vi "SP Append Filter Skirt Limit Waveform.vi"(4 "Limit Format":T2, 5 "Number of Points":i32, 6 "Measured Parameter":T3={"Stimulus Port"=1, "Response Port"=1} {"Stimulus Port" min=1 step=1; "Response Port" min=1 step=1}, 7 "Attribute Name (NI_ChannelName)":string="NI_ChannelName", 8 "error in (no error)":errorcluster, 9 "Limits Pass/Fail":cluster{"Upper Pass?":bool, "Lower Pass?":bool}, 10 "Upper and Lower Limits":T1={"Upper Limit"={"F0"=500.0, "dF"=1.0, "Formatted Values"=[-6.0, -6.0, -6.0, -6.0, -6.0, -6.0, -5.0, -4.0, -3.0, -2.0, -1.0017226002993769, -0.8636286738753696, -1.012432061728755, -0.8135188671805874, -1.084383696215112, -1.192695586219516, -0.8228939725524264, -1.1588169801015764, -1.0069715761898415, -0.8118111488159718, -0.9516999033989667, -1.0842662636672022, -1.0261931083967077, -0.816874162233468, -0.8335770068326294, -1.1794529347576463, -1.1032959879886735, -1.197742447623333, -0.9631229100196212, -0.9908453124177325, -0.9835470980893588, -1.10217991844936, -0.8956607286257672, -0.8794782872077156, -0.9013683651609963, -1.0772188731817596, -0.992723355191172, -0.9536275499498994, -0.9874327685983141, -0.921963653527827, -0.8848787728556787, -1.1874980208218, -0.996957511881206, -0.9972503730309241, -0.8866139538542095, -1.07344181331393, -0.881559772443858, -1.0112449407130875, -0.9865384477979471, -0.9901446738263366, -1.1718630063784758, -0.9951725256878827, -0.931778781153855, -0.9846289731021831, -0.851763264124267, -0.9086965469391421, -0.8349429101974368, -0.8383742350256687, -1.106571816484691, -0.9554005266395742, -0.9376822403043366, -1.131287512516927, -1.0382288806403288, -0.917054052988136, -0.9489467877812984, -0.9264227759143271, -1.0918690925892351, -1.1668737446636852, -1.0021735712381068, -1.1541225361979714, -1.1931131329605709, -0.8730502330378824, -0.850411285659811, -1.137775166801135, -1.1870586525662095, -1.0926571181161528, -1.118993526927924, -1.1211410787283602, -0.8920697041785735, -0.888430731015914, -1.0656600076605476, -1.1666787859795846, -1.0713340188424678, -0.8625910088884297, -1.1434360227216422, -0.9217710376784376, -1.1218396445954617, -0.9558195687190933, -1.1773692443654946, -1.0827782751424972, -1.1567791336122029, -0.8684407402614696, -0.8177845157195978, -0.9040657051180614, -0.9313557288389804, -1.0236831450620423, -1.050426714979035, -0.8344777069605718, -0.8274082929927138, -1.1990080831766776, -1.0947798998491134, -1.1963114865246718, -1.0016247375583676, -1.0877110100652403, -1.1556028882288836, -1.1918380581525247, -0.9751292214691399, -0.8884133044813358, -1.0347444321214612, -0.9445125246491541, -2.0, -3.0, -4.0, -5.0, -6.0, -6.0, -6.0, -6.0, -6.0, -6.0]}, "Lower Limit"={"F0"=500.0, "dF"=1.0, "Formatted Values"=[-6.0, -6.0, -6.0, -6.0, -6.0, -6.0, -5.0, -4.0, -3.0, -2.0, -1.0017226002993769, -0.8636286738753696, -1.012432061728755, -0.8135188671805874, -1.084383696215112, -1.192695586219516, -0.8228939725524264, -1.1588169801015764, -1.0069715761898415, -0.8118111488159718, -0.9516999033989667, -1.0842662636672022, -1.0261931083967077, -0.816874162233468, -0.8335770068326294, -1.1794529347576463, -1.1032959879886735, -1.197742447623333, -0.9631229100196212, -0.9908453124177325, -0.9835470980893588, -1.10217991844936, -0.8956607286257672, -0.8794782872077156, -0.9013683651609963, -1.0772188731817596, -0.992723355191172, -0.9536275499498994, -0.9874327685983141, -0.921963653527827, -0.8848787728556787, -1.1874980208218, -0.996957511881206, -0.9972503730309241, -0.8866139538542095, -1.07344181331393, -0.881559772443858, -1.0112449407130875, -0.9865384477979471, -0.9901446738263366, -1.1718630063784758, -0.9951725256878827, -0.931778781153855, -0.9846289731021831, -0.851763264124267, -0.9086965469391421, -0.8349429101974368, -0.8383742350256687, -1.106571816484691, -0.9554005266395742, -0.9376822403043366, -1.131287512516927, -1.0382288806403288, -0.917054052988136, -0.9489467877812984, -0.9264227759143271, -1.0918690925892351, -1.1668737446636852, -1.0021735712381068, -1.1541225361979714, -1.1931131329605709, -0.8730502330378824, -0.850411285659811, -1.137775166801135, -1.1870586525662095, -1.0926571181161528, -1.118993526927924, -1.1211410787283602, -0.8920697041785735, -0.888430731015914, -1.0656600076605476, -1.1666787859795846, -1.0713340188424678, -0.8625910088884297, -1.1434360227216422, -0.9217710376784376, -1.1218396445954617, -0.9558195687190933, -1.1773692443654946, -1.0827782751424972, -1.1567791336122029, -0.8684407402614696, -0.8177845157195978, -0.9040657051180614, -0.9313557288389804, -1.0236831450620423, -1.050426714979035, -0.8344777069605718, -0.8274082929927138, -1.1990080831766776, -1.0947798998491134, -1.1963114865246718, -1.0016247375583676, -1.0877110100652403, -1.1556028882288836, -1.1918380581525247, -0.9751292214691399, -0.8884133044813358, -1.0347444321214612, -0.9445125246491541, -2.0, -3.0, -4.0, -5.0, -6.0, -6.0, -6.0, -6.0, -6.0, -6.0]}}, 11 "Waveforms in":waveform(dbl)[](array[waveform])) -> (0 "error out":errorcluster, 3 "Waveforms out":waveform(dbl)[](array[waveform]))   [LabVIEW 2011]
uses:
  TypeDefs/SP Parameter.ctl
  TypeDefs/SP Format.ctl
  TypeDefs/SP Channel Type.ctl
  Channel Test Status Enumeration.ctl
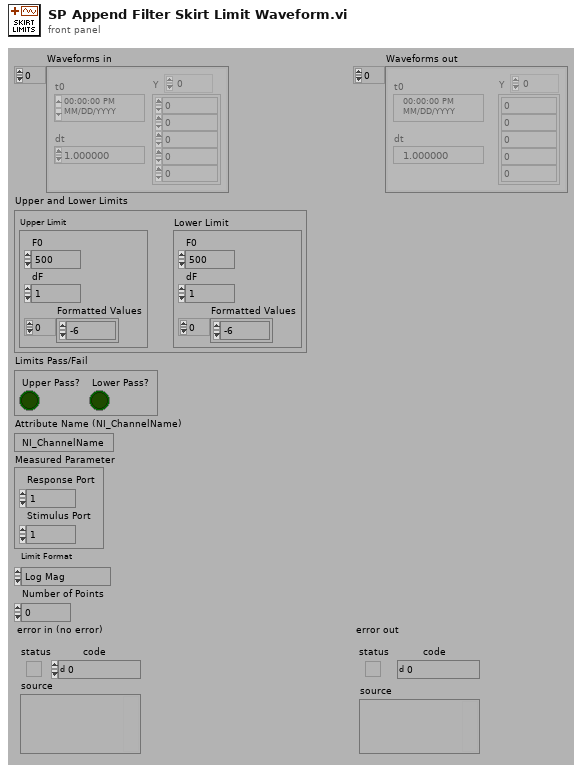
[diagram p1: front panel]
types:
  T1 = cluster{"Upper Limit":cluster{"F0":dbl, "dF":dbl, "Formatted Values":dbl[]}, "Lower Limit":cluster{"F0":dbl, "dF":dbl, "Formatted Values":dbl[]}}
  T2 = typedef "SP Format.ctl" = enum16{"Log Mag", "Lin Mag", "SWR", "Phase", "Expanded Phase", "Delay", "Insertion Loss", "Isolation", "Return Loss"}
  T3 = typedef "SP Parameter.ctl" = cluster{"Stimulus Port":i8, "Response Port":i8}
  T4 = typedef "SP Channel Type.ctl" = enum16{"Frequency", "Data", "Limit", "Adapter", "Memory", "Value", "Value Limit"}
  T5 = typedef "Channel Test Status Enumeration.ctl" = enum16{"Fail", "Pass", "Abort", "Error", "Done", "Pass by Sample", "Fail by Sample", "Pass Override", "Fail Override", "Not Tested"}
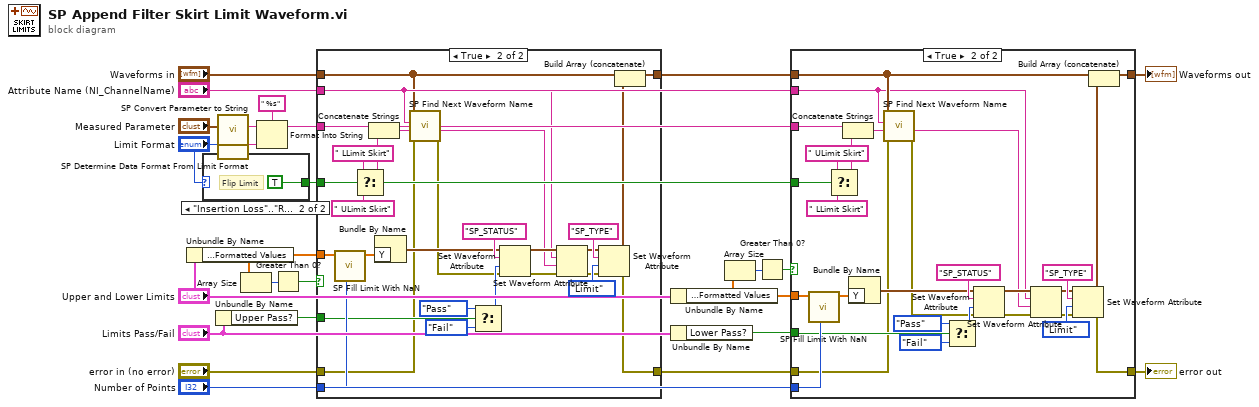
[diagram p0: block diagram]
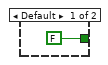
[diagram p3: hidden frame]
diagram:
  n1 = Unbundle By Name("Upper and Lower Limits") -> ("Upper Limit.Formatted Values"=w12:dbl[])
  n2 = case shown="\"Insertion Loss\"..\"Return Loss\"" "Limit Format" {
    tunnel: [FALSE TRUE] -> w9
    frame Default {
    }
    frame "Insertion Loss".."Return Loss" {
      # "Flip Limit"
    }
  }
  n3 = Unbundle By Name("Limits Pass/Fail") -> ("Upper Pass?"=w18:bool)
  n4 = call "SP Convert Parameter to String.vi"("Parameter"="Measured Parameter") -> ("Parameter String"=w15:string)  [unwired: 10 out]
  n5 = call "SP Determine Data Format From Limit Format.vi"("Limit Format"="Limit Format") -> ("Format String"=w14:string)
  n6 = Array Size(array=w12) -> (size(s)=w23:i32)
  n7 = Format Into String(format string=" %s", initial string=w15, w14) -> (resulting string=w10:string)  [unwired: 1 in, 1 out]
  n8 = Greater Than 0?(x=w23) -> (x > 0?=w21:bool)
  n9 = case shown="True" w21 {
    tunnel: "Waveforms in" -> [w28 w35]
    tunnel: "error in (no error)" -> [w29 w31]
    tunnel: [w29 w38] -> w4
    tunnel: "Attribute Name (NI_ChannelName)" -> [_ w33]
    tunnel: w12 -> [_ w53]
    tunnel: w10 -> [_ w58]
    tunnel: [w28 w36] -> w3
    tunnel: w18 -> [_ w47]
    tunnel: w9 -> [_ w54]
    tunnel: "Number of Points" -> [_ w51]
    frame False {
    }
    frame True {
      n10 = call "SP Fill Limit With NaN.vi"("Number of Points"=w51, "Limit"=w53) -> ("Filled Limit"=w52:dbl[])  [unwired: 9 out]
      n11 = Select(t=" LLimit Skirt", s=w54, f=" ULimit Skirt") -> (s? t:f=w55:string)
      n12 = Concatenate Strings(w58, w55) -> (w34:string)
      n13 = Bundle By Name("Y"=w52) -> (w45:waveform(dbl))  [unwired: 1 out]
      n14 = call "SP Find Next Waveform Name.vi"("error in (no error)"=w31, "Prospective Base Name"=w34, "Attribute Name (NI_ChannelName)"=w33, "Waveforms in"=w35) -> ("error out"=w30:errorcluster, "Channel Name"=w32:string)  [unwired: 6 in]
      n15 = Select(t=Channel_Test_Status_Enumeration."Pass" ("Channel Status Enumeration"), s=w47, f=Channel_Test_Status_Enumeration."Fail" ("Channel Status Enumeration")) -> (s? t:f=w46:T5)
      n16 = Set Waveform Attribute(4:w30, 5:w46, 6:"SP_STATUS", 7:w45) -> (0:w39:errorcluster, 3:w42:waveform(dbl))  [unwired: 1 out]
      n17 = Set Waveform Attribute(4:w39, 5:w32, 6:w33, 7:w42) -> (0:w40:errorcluster, 3:w41:waveform(dbl))  [unwired: 1 out]
      n18 = Set Waveform Attribute(4:w40, 5:SP_Channel_Type."Limit" ("Channel Type"), 6:"SP_TYPE", 7:w41) -> (0:w38:errorcluster, 3:w37:waveform(dbl))  [unwired: 1 out]
      n19 = Build Array (concatenate)(w35, w37) -> (w36:waveform(dbl)[])
    }
  }
  n20 = Unbundle By Name("Upper and Lower Limits") -> ("Lower Limit.Formatted Values"=w6:dbl[])
  n21 = Unbundle By Name("Limits Pass/Fail") -> ("Lower Pass?"=w7:bool)
  n22 = Array Size(array=w6) -> (size(s)=w20:i32)
  n23 = Greater Than 0?(x=w20) -> (x > 0?=w8:bool)
  n24 = case shown="True" w8 {
    tunnel: w3 -> [w59 w66]
    tunnel: w4 -> [w60 w62]
    tunnel: [w60 w69] -> w1
    tunnel: "Attribute Name (NI_ChannelName)" -> [_ w64]
    tunnel: w6 -> [_ w84]
    tunnel: w10 -> [_ w89]
    tunnel: [w59 w67] -> w2
    tunnel: w7 -> [_ w78]
    tunnel: w9 -> [_ w85]
    tunnel: "Number of Points" -> [_ w82]
    frame False {
    }
    frame True {
      n25 = call "SP Fill Limit With NaN.vi"("Number of Points"=w82, "Limit"=w84) -> ("Filled Limit"=w83:dbl[])  [unwired: 9 out]
      n26 = Select(t=" ULimit Skirt", s=w85, f=" LLimit Skirt") -> (s? t:f=w86:string)
      n27 = Concatenate Strings(w89, w86) -> (w65:string)
      n28 = Bundle By Name("Y"=w83) -> (w76:waveform(dbl))  [unwired: 1 out]
      n29 = call "SP Find Next Waveform Name.vi"("error in (no error)"=w62, "Prospective Base Name"=w65, "Attribute Name (NI_ChannelName)"=w64, "Waveforms in"=w66) -> ("error out"=w61:errorcluster, "Channel Name"=w63:string)  [unwired: 6 in]
      n30 = Select(t=Channel_Test_Status_Enumeration."Pass" ("Channel Status Enumeration"), s=w78, f=Channel_Test_Status_Enumeration."Fail" ("Channel Status Enumeration")) -> (s? t:f=w77:T5)
      n31 = Set Waveform Attribute(4:w61, 5:w77, 6:"SP_STATUS", 7:w76) -> (0:w70:errorcluster, 3:w73:waveform(dbl))  [unwired: 1 out]
      n32 = Set Waveform Attribute(4:w70, 5:w63, 6:w64, 7:w73) -> (0:w71:errorcluster, 3:w72:waveform(dbl))  [unwired: 1 out]
      n33 = Set Waveform Attribute(4:w71, 5:SP_Channel_Type."Limit" ("Channel Type"), 6:"SP_TYPE", 7:w72) -> (0:w69:errorcluster, 3:w68:waveform(dbl))  [unwired: 1 out]
      n34 = Build Array (concatenate)(w66, w68) -> (w67:waveform(dbl)[])
    }
  }
  "Waveforms out" <- w2
  "error out" <- w1
